vi "tx_make_plots.vi"(0 "waveform":T2={"t0"=0.0, "dt"=1.0, "Y"=[]} {"Y" format="%.3f"; "dt" format="%^.2e"; "t0" format="%.4f"}, 5 "Y":cdb[](array[numeric]), 7 "eye length":i32=1, 9 "symbol rate (Hz)":dbl=1.0 format="%.2f", 11 "I/Q (I)":enum16{"I", "Q"}(ring)) -> (4 "eye diagram":cluster{"t0":dbl, "dt":dbl, "Y":dbl[]}[](array[cluster]) {"Y" format="%.2f"; "dt" format="%.2f"; "t0" format="%.2f"}, 6 "constellation graph":T1(array[cluster]) {"oversampled data" format="%.2f"; "constellation" format="%.2f"}, 8 "IQ data (complex) out":cluster{"t0":dbl, "dt":dbl, "Y":cdb[]} {"Y" format="%.2f"; "dt" format="%.2f"; "t0" format="%.2f"}, 10 "r":dbl[](array[numeric]), 13 "I component":waveform(dbl), 14 "Q component":waveform(dbl), 15 "theta":dbl[](array[numeric]))   [LabVIEW 2012]
uses:
  <vilib>/addons/Modulation/Analog/controls/Complex Data Waveform.ctl
  <vilib>/Analysis/2dsp.llb/Complex FFT.vi
  <vilib>/addons/Modulation/Digital/General/MT Format Eye Diagram (complex).vi
  <vilib>/addons/Modulation/niDMT.lvlib
  <vilib>/addons/Modulation/niAMT.lvlib
  <vilib>/Analysis/NI_AALPro.lvlib
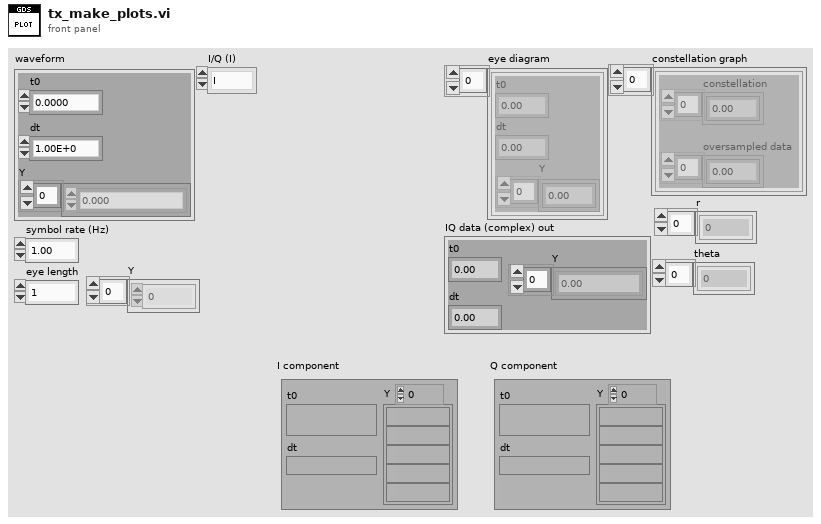
[diagram p1: front panel]
types:
  T1 = cluster{"constellation":dbl[], "oversampled data":dbl[]}[]
  T2 = typedef "niAMT.lvlib/Complex Data Waveform.ctl" = cluster{"t0":dbl, "dt":dbl, "Y":cdb[]}
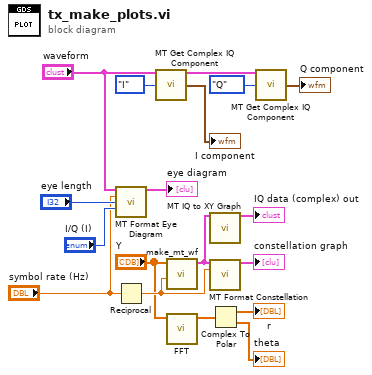
[diagram p0: block diagram]
diagram:
  n1 = call-poly <vilib>:"MT Format Eye Diagram.vi"("waveform"="waveform", "symbol rate (Hz)"="symbol rate (Hz)", "eye length"="eye length", "I/Q (I)"="I/Q (I)") -> ("eye diagram"=→"eye diagram":cluster{"t0":dbl, "dt":dbl, "Y":dbl[]}[])  [unwired: 10 in, 1 out]
  n2 = Reciprocal(x="symbol rate (Hz)") -> (1/x=w13:dbl)
  n3 = call <vilib>:"MT Get Complex IQ Component.vi"("IQ data (complex) in"="waveform", "component choice"=enum16{"I", "Q", "Magnitude", "Phase"}."I") -> ("IQ data (complex) out"=w11:cluster{"t0":dbl, "dt":dbl, "Y":cdb[]}, "CE component"=→"I component":waveform(dbl))  [unwired: 11 in, 1 out]
  n4 = call "make_mt_wf.vi"("dt"=w13, "Y"="Y") -> ("output MT waveform"=w14:cluster{"t0":dbl, "dt":dbl, "Y":cdb[]})  [unwired: 9 in]
  n5 = call-poly <vilib>:"FFT.vi"("X"="Y") -> ("FFT {X}"=w3:cdb[])  [unwired: 9 in, 1 out]
  n6 = call <vilib>:"MT IQ to XY Graph.vi"("IQ data (complex) in"=w14) -> ("IQ data (complex) out"=→"IQ data (complex) out":cluster{"t0":dbl, "dt":dbl, "Y":cdb[]})  [unwired: 12 in, 2 out]
  n7 = call <vilib>:"MT Format Constellation.vi"("waveform"=w14, "samples per symbol"=w13) -> ("constellation graph"=→"constellation graph":T1)  [unwired: 12 in, 1 out]
  n8 = Complex To Polar(r * e^(i*theta)=w3) -> (r=→"r":dbl[], theta=→"theta":dbl[])
  n9 = call <vilib>:"MT Get Complex IQ Component.vi"("IQ data (complex) in"=w11, "component choice"=enum16{"I", "Q", "Magnitude", "Phase"}."Q") -> ("CE component"=→"Q component":waveform(dbl))  [unwired: 11 in, 2 out]
